vi "Establish Connection - Client.vi"(0 "server address":string="127.0.0.1", 3 "error in (no error)":errorcluster) -> (7 "Message from Server":string, 8 "Connection Established?":bool, 10 "No error":errorcluster)   [LabVIEW 2020]
doc: "Tests ports in direction of cliend to server"
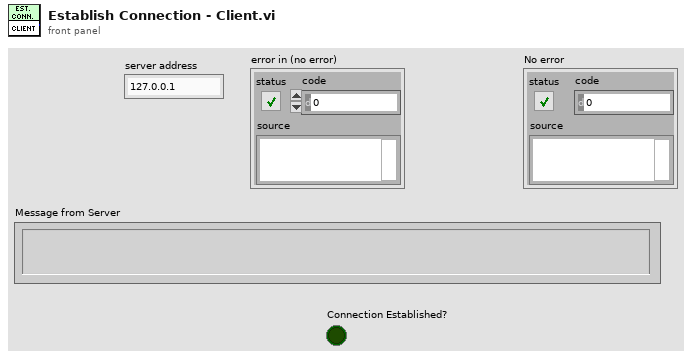
[diagram p1: front panel]
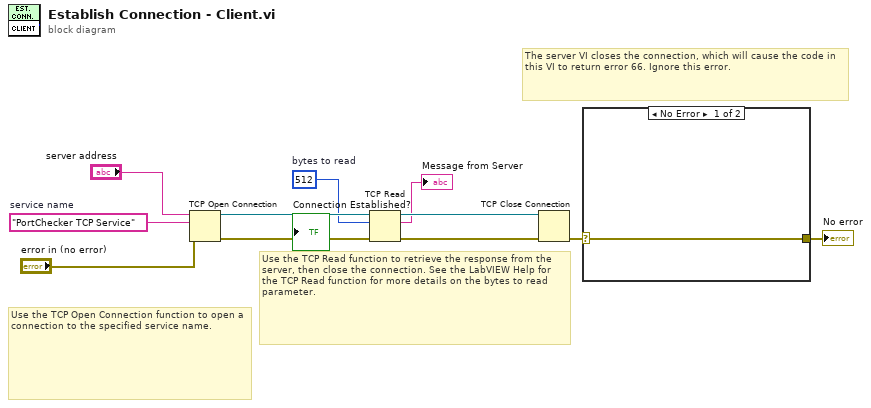
[diagram p0: block diagram]
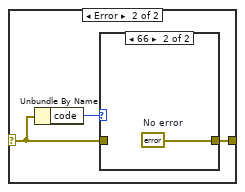
[diagram p2: hidden frame]
diagram:
  w4 = 512  # bytes to read
  w5 = "PortChecker TCP Service"  # service name
  # "The server VI closes the connection, which will cause the code in this VI to return error 66. Ignore this error."
  # "Use the TCP Open Connection function to open a connection to the specified service name."
  # "Use the TCP Read function to retrieve the response from the server, then close the connection. See the LabVIEW Help for the TCP Read function for more details on the bytes to read parameter."
  n1 = TCP Open Connection(address="server address", remote port or service name=w5, error in (no error)="error in (no error)") -> (connection ID=w10:refnum<k5>, error out=w11:errorcluster)  [unwired: 2 in]
  n2 = TCP Read(connection ID=w10, bytes to read=w4, error in (no error)=w11) -> (connection ID out=w9:refnum<k5>, data out=→"Message from Server":string, error out=w8:errorcluster)  [unwired: 2 in]
  n3 = TCP Close Connection(connection ID=w9, error in (no error)=w8) -> (error out=w3:errorcluster)  [unwired: 1 in, 1 out]
  n4 = case shown="No Error" w3 {
    selector: w3 -> [w12 w14]
    tunnel: [w12 w13] -> w2
    frame No Error {
    }
    frame Error {
      n5 = Unbundle By Name(w14) -> ("code"=w15:i32)
      n6 = case shown="66" w15 {
        tunnel: w14 -> [w16 _]
        tunnel: [w16 w17] -> w13
        frame Default {
        }
        frame 66 {
          w17 = errorcluster {"status"=FALSE, "code"=0, "source"=""}  # No error
        }
      }
    }
  }
  "No error" <- w2
